vi "randomDataBase64url.vi"(11 "length":i32) -> (3 "base64 string":string)   [LabVIEW 2020, in "Netatmo-WeatherStation.lvlib"]
uses:
  Netatmo-WeatherStation.lvlib
  <vilib>/numeric/Random Number (Range) I64.vi
  <vilib>/numeric/sub_Random U32.vi
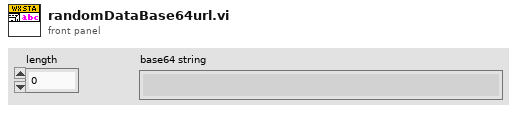
[diagram p1: front panel]
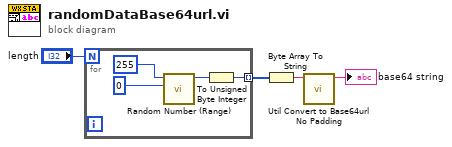
[diagram p0: block diagram]
diagram:
  n1 = for {
    N: "length" -> [_]
    tunnel: [w5] -> w1 mode=indexing
    n2 = call-poly <vilib>:"Random Number (Range).vi"("lower bound (-100)"=i64 0, "upper bound (100)"=i64 255) -> ("number"=w6:i64)  [unwired: 9 in]
    n3 = To Unsigned Byte Integer(number=w6) -> (unsigned 8bit integer=w5:u8)
  }
  n4 = Byte Array To String(unsigned byte array=w1) -> (string=w3:string)
  n5 = call "Util Convert to Base64url No Padding.vi"("String (hex display)"=w3) -> ("Base64url String"=→"base64 string":string)  [unwired: 10 in]
